vi "set_overlay.vi"(8 "error in (no error)":errorcluster, 9 "raw channel index":i32, 10 "palette in":cluster{"Red":u8, "Green":u8, "Blue":u8}[](array[cluster]), 11 "DisplayDL090216 in":refnum<class "DisplayDL090216.lvclass">) -> (0 "error out":errorcluster, 3 "DisplayDL090216 out":refnum<class "DisplayDL090216.lvclass">)   [LabVIEW 2010, in "DisplayDL090216.lvclass"]
uses:
  DisplayDL090216.lvclass
  DisplayDL090216.lvclass/DisplayDL090216.ctl
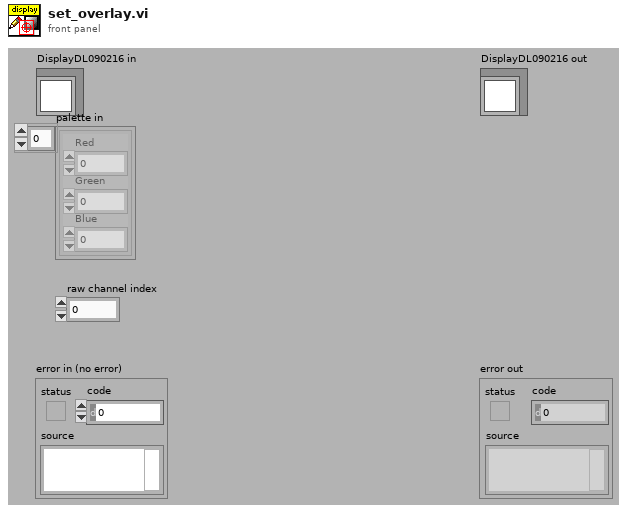
[diagram p1: front panel]
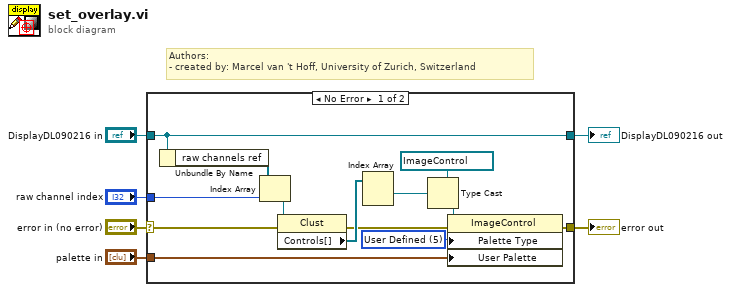
[diagram p0: block diagram]
diagram:
  # "Authors: \n- created by: Marcel van 't Hoff, University of Zurich, Switzerland"
  n1 = case shown="No Error" "error in (no error)" {
    selector: "error in (no error)" -> [w12 w21]
    tunnel: [w11 w21] -> w5
    tunnel: [w14 w20] -> w3
    tunnel: "DisplayDL090216 in" -> [w14 w20]
    tunnel: "palette in" -> [w9 _]
    tunnel: "raw channel index" -> [w7 _]
    frame No Error {
      w8 = u32 5 items=["Grayscale", "Binary", "Gradient", "Rainbow", "Temperature", "User Defined"] ("Palette:Palette Type")
      n2 = Unbundle By Name(w14) -> ("raw channels ref"=w18:refnum<vi>[])
      n3 = Index Array(array=w18, index=w7) -> (element=w19:refnum<vi>)
      n4 = property class="Clust"(reference=w19, error in=w12) -> (error out=w13:errorcluster, "Controls[]"=w15:refnum<vi>[])  [unwired: 1 out]
      n5 = Index Array(array=w15) -> (element #1=w16:refnum<vi>)  [unwired: 2 in, 1 out]
      n6 = Type Cast(type=refnum<vi> refnum ("histogram out"), x=w16) -> (*(type *) &x=w10:refnum<vi>)
      n7 = property class="ImageControl"(reference=w10, error in=w13, "Palette Type"=w8, "User Palette"=w9) -> (error out=w11:errorcluster)  [unwired: 1 out]
    }
    frame Error {
    }
  }
  "error out" <- w5
  "DisplayDL090216 out" <- w3
